vi "pulse creation 2nd.vi"(8 "error in":errorcluster, 11 "chopper width(usec)":u32=400) -> (0 "error out":errorcluster, 2 "mean":dbl format="%0.2f", 3 "Waveform Graph":dbl[](graph))   [LabVIEW 2016]
doc: "Sends a pulse to the chopper. Then the stable current is measured in the offset cup"
uses:
  <vilib>/DAQmx/write.llb/DAQmx Write (Digital Wfm 1Chan NSamp).vi
  <vilib>/DAQmx/read.llb/DAQmx Read (Analog 1D DBL 1Chan NSamp).vi
  <vilib>/DAQmx/miscellaneous.llb/DAQmx Fill In Error Info.vi
  <vilib>/Waveform/DWDTOps.llb/DWDT Uncompress Digital.vi
  <resource>/objmgr/daqmx.rc
panel:
  out "data":dbl[][](array[numeric]) format="%0.2f"
  out "subarray 3":dbl[](array[numeric])
  out "subarray 2":dbl[](array[numeric])
  out "subarray":dbl[](array[numeric])
  out "error out 3":errorcluster
  out "sum":dbl
  out "stop? 2":bool
  out "stop?":bool
  out "error out 2":errorcluster
  out "error out 6":errorcluster
  out "error out 5":errorcluster
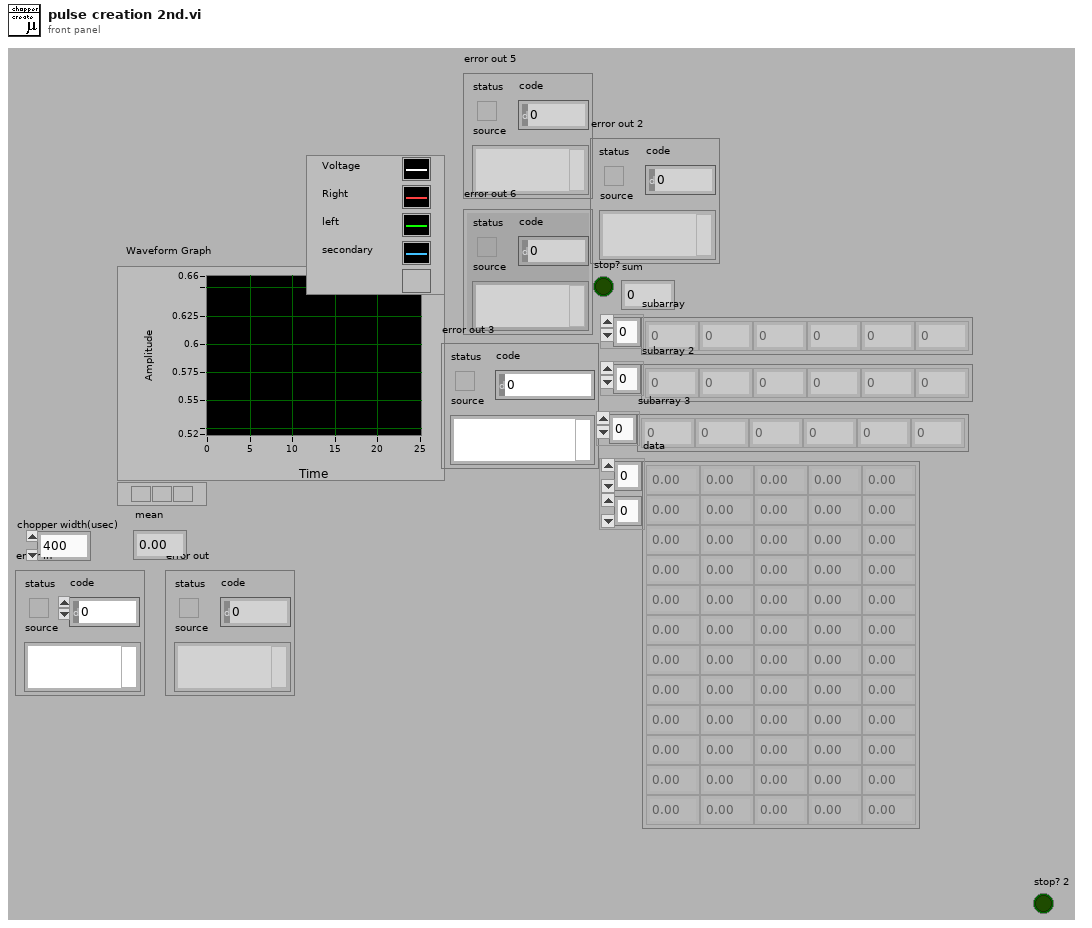
[diagram p1: front panel]
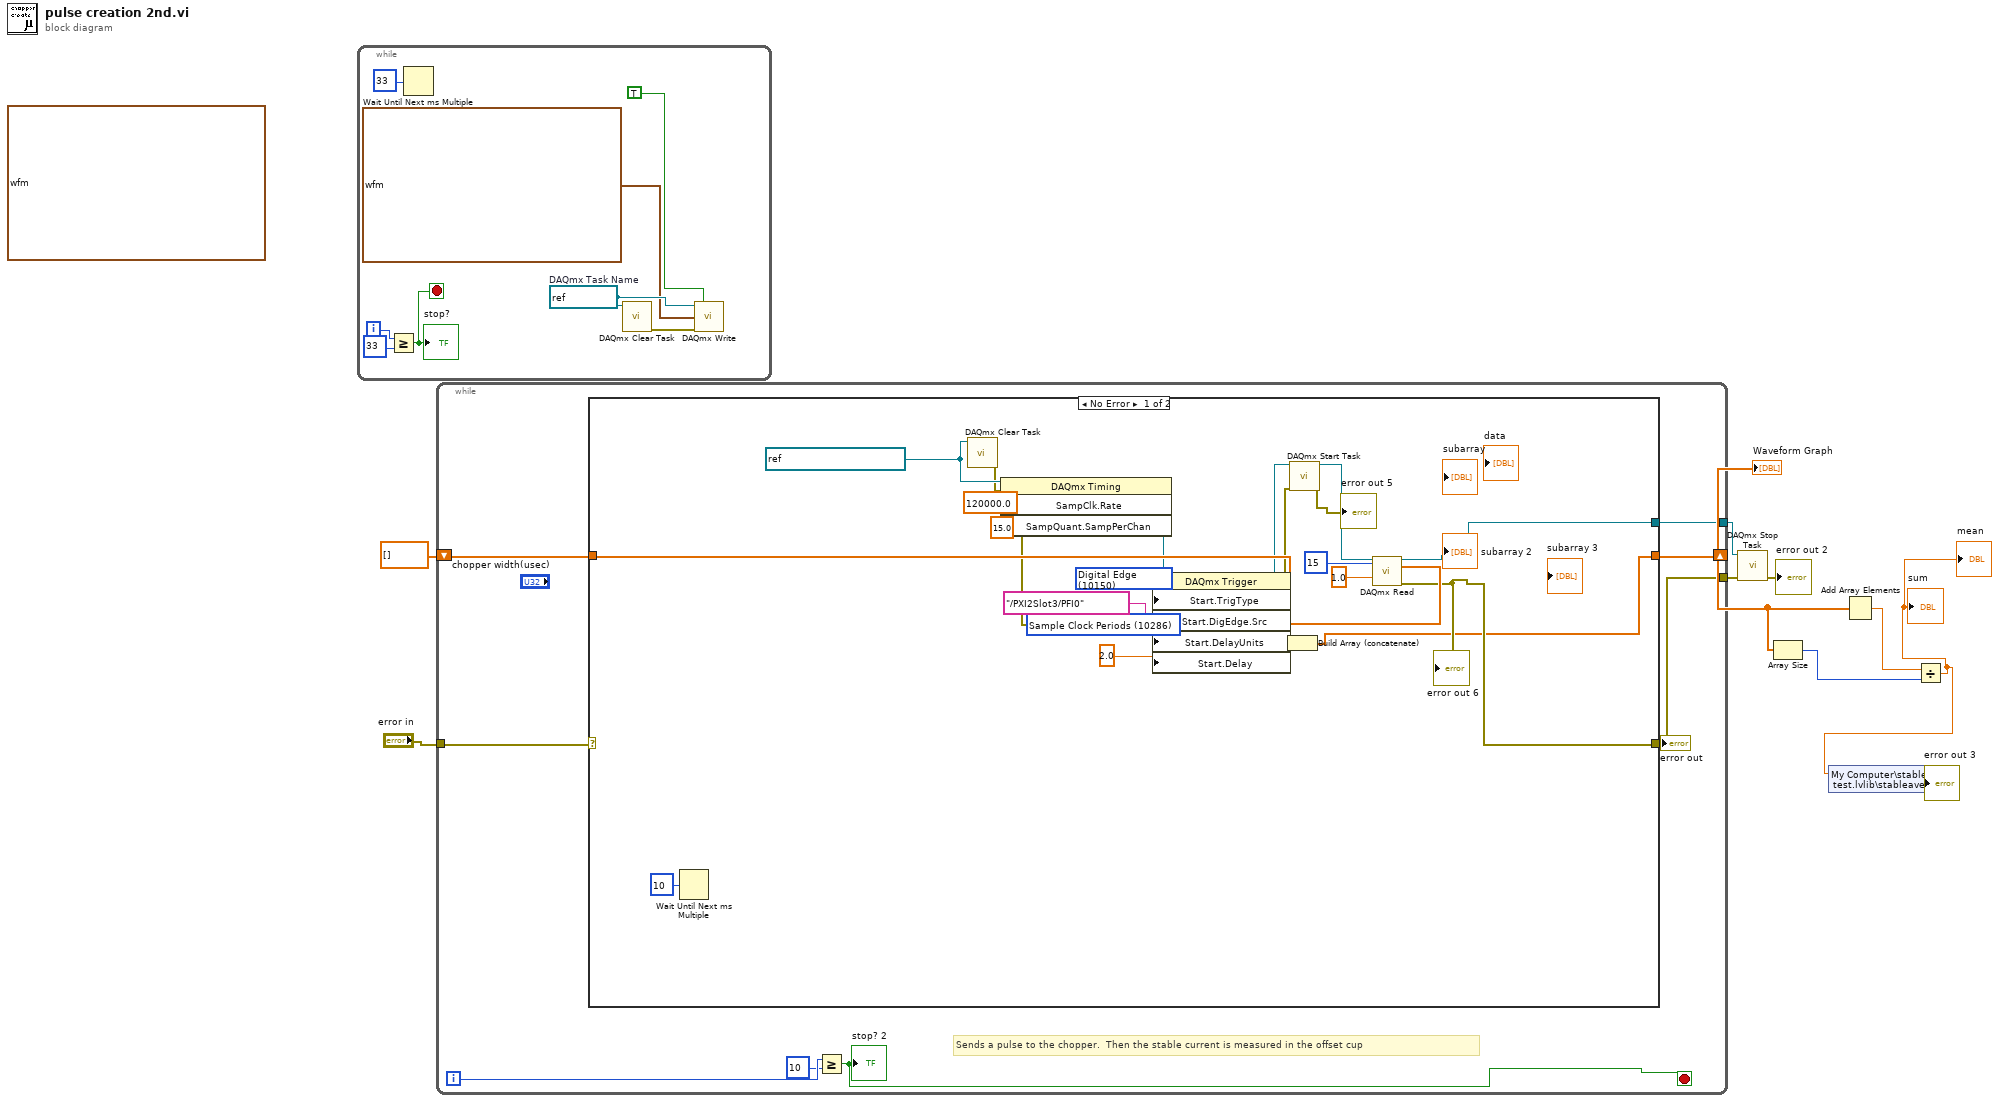
[diagram p0: block diagram]
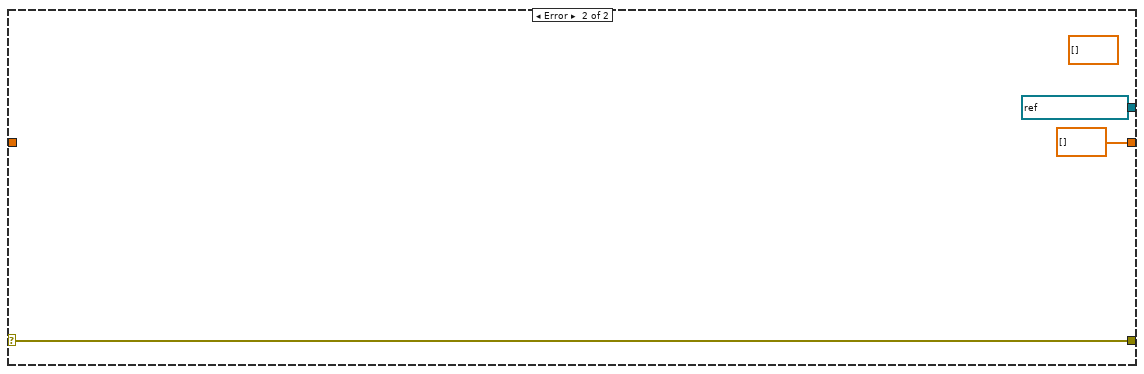
[diagram p2: hidden frame]
diagram:
  (unwired) digitalwaveform {"t0"=timestamp(0 s since 1904-01-01), "dt"=0.0001, "Y"={"transitions"=[], "data"=array1150x16[18400 elements]}} ("digital waveform")
  n1 = while {
    i -> [w15]
    stop <- w13 stop-if-true
    w17 = refnum<k21> "chop2"  # DAQmx Task Name
    n2 = Greater Or Equal?(x=w15, y=33) -> (x >= y?=w13:bool)
    "stop?" <- w13
    n3 = Wait Until Next ms Multiple(millisecond multiple=u32 33) -> ()  [unwired: 1 out]
    n4 = call <vilib>:"DAQmx Clear Task.vi"("task in"=w17) -> ("error out"=w18:errorcluster)  [unwired: 14 in]
    n5 = call-poly <vilib>:"DAQmx Write.vi"("task/channels in"=w17, "auto start"=TRUE, "data"=digitalwaveform {"t0"=timestamp(0 s since 1904-01-01), "dt"=0.0001, "Y"={"transitions"=[], "data"=array1150x16[18400 elements]}} ("digital waveform"), "error in"=w18) -> ()  [unwired: 9 in, 3 out]
  }
  n6 = while {
    tunnel: "error in" -> [w26]
    tunnel: [w25] -> w9
    tunnel: [w24] -> w8
    shift-right: [w23] -> w1
    shift-left: dbl[] [] -> [w22]
    i -> [w20]
    stop <- w21 stop-if-true
    # "Sends a pulse to the chopper.  Then the stable current is measured in the offset cup"
    n7 = case shown="No Error" w26 {
      selector: w26 -> [_ w51]
      tunnel: [w32 w51] -> w24
      tunnel: [w42 refnum<k21> "sum current" ("task out")] -> w25
      tunnel: [w29 dbl[] []] -> w23
      tunnel: w22 -> [w41 _]
      frame No Error {
        w28 = 10286 items=["Sample Clock Periods"=10286, "Seconds"=10364, "Ticks"=10304] ("Start.DelayUnits")
        w40 = refnum<k21> "secondary current" ("task/channels in")
        w43 = 10150 items=["Analog Edge"=10099, "Digital Edge"=10150, "Digital Pattern"=10398, "Analog Window"=10103, "None"=10230] ("Start.TrigType")
        n8 = Wait Until Next ms Multiple(millisecond multiple=u32 10) -> ()  [unwired: 1 out]
        n9 = call <vilib>:"DAQmx Clear Task.vi"("task in"=w40) -> ("error out"=w38:errorcluster)  [unwired: 14 in]
        n10 = property class="DAQmx Timing"(reference=w40, error in=w38, "SampClk.Rate"=120000.0, "SampQuant.SampPerChan"=15.0 ("SampClk.Rate")) -> (reference out=w39:refnum<k21>, error out=w36:errorcluster)
        n11 = property class="DAQmx Trigger"(reference=w39, error in=w36, "Start.TrigType"=w43, "Start.DigEdge.Src"=tag "/PXI2Slot3/PFI0", "Start.DelayUnits"=w28, "Start.Delay"=2.0) -> (reference out=w37:refnum<k21>, error out=w35:errorcluster)
        n12 = call <vilib>:"DAQmx Start Task.vi"("task/channels in"=w37, "error in"=w35) -> ("task out"=w48:refnum<k21>, "error out"=→"error out 5":errorcluster)  [unwired: 12 in]
        n13 = call-poly <vilib>:"DAQmx Read.vi"("task/channels in"=w48, "number of samples per channel"=15, "timeout"=1.0) -> ("task out"=w42:refnum<k21>, "data"=w33:dbl[], "error out"=w32:errorcluster)  [unwired: 10 in]
        "error out 6" <- w32
        n14 = Build Array (concatenate)(w41, w33) -> (w29:dbl[])
      }
      frame Error {
        (unwired) dbl[] []
      }
    }
    "error out" <- w24
    n15 = Greater Or Equal?(x=w20, y=10) -> (x >= y?=w21:bool)
    "stop? 2" <- w21
  }
  "Waveform Graph" <- w1
  n16 = call <vilib>:"DAQmx Stop Task.vi"("task/channels in"=w9, "error in"=w8) -> ("error out"=→"error out 2":errorcluster)  [unwired: 12 in, 1 out]
  n17 = Array Size(array=w1) -> (size(s)=w2:i32)
  n18 = Add Array Elements(numeric array=w1) -> (sum=w5:dbl)
  n19 = Divide(x=w5, y=w2) -> (x/y=w3:dbl)
  "sum" <- w3
  "mean" <- w3
  n20 = shared-variable "My Computer\\stable test.lvlib\\stableave"(w3) -> (error out=→"error out 3":errorcluster)  [unwired: 1 in]
